vi "Append Text.vi"(7 "Style":T1={"Name"="Default", "Font"={"Name"="Calibri", "Size"=12, "Bold"=FALSE, "Italic"=FALSE, "Underline"=18, "Strike"=FALSE, "Color"=0, "Alignment"=1}} {"Font"."Alignment" items=["LEFT"=1, "CENTER"=2, "RIGHT"=3, "BOTH"=4, "MEDIUM_KASHIDA"=5, "DISTRIBUTE"=6, "NUM_TAB"=7, "HIGH_KASHIDA"=8, "LOW_KASHIDA"=9, "THAI_DISTRIBUTE"=10]; "Font"."Underline" items=["Single"=1, "Words"=2, "Double"=3, "Thick"=4, "Dotted"=5, "DottedHeavy"=6, "Dash"=7, "DashedHeavy"=8, "DashLong"=9, "DashLongHeavy"=10, "DotDash"=11, "DashDotHeavy"=12, "DotDotDash"=13, "DashDotDotHeavy"=14, "Wave"=15, "WavyHeavy"=16, "WavyDouble"=17, "None"=18]}, 8 "error in (no error)":errorcluster, 10 "Text":string, 11 "Document in":refnum<class "Document.lvclass">) -> (0 "error out":errorcluster, 3 "Document out":refnum<class "Document.lvclass">)   [LabVIEW 2017, in "LabVIEW NPOI.lvlib" / "Document.lvclass"]
uses:
  Document.lvclass
  Styles/Style--cluster.ctl
  Styles/Font--cluster.ctl
  Styles/Underline--ring.ctl
  Styles/Alignment--ring.ctl
  Styles/Styles.lvlib
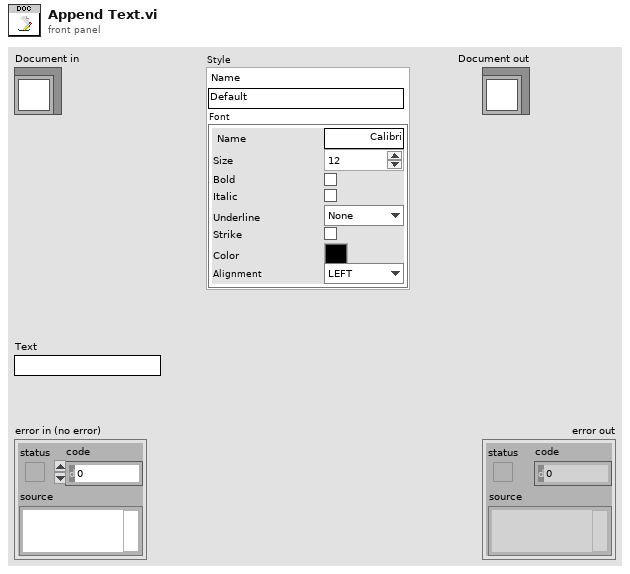
[diagram p1: front panel]
types:
  T1 = typedef "Styles.lvlib/Style--cluster.ctl" = cluster{"Name":string, "Font":T2}
  T2 = typedef "Styles.lvlib/Font--cluster.ctl" = cluster{"Name":string, "Size":i32, "Bold":bool, "Italic":bool, "Underline":T3, "Strike":bool, "Color":u32, "Alignment":T4}
  T3 = typedef "Styles.lvlib/Underline--ring.ctl" = i32
  T4 = typedef "Styles.lvlib/Alignment--ring.ctl" = i32
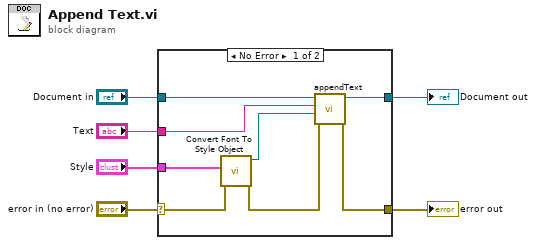
[diagram p0: block diagram]
diagram:
  n1 = case shown="No Error" "error in (no error)" {
    selector: "error in (no error)" -> [w9 w16]
    tunnel: [w7 w16] -> w5
    tunnel: [w12 w15] -> w3
    tunnel: "Document in" -> [w13 w15]
    tunnel: "Style" -> [w14 _]
    tunnel: "Text" -> [w10 _]
    frame No Error {
      n2 = call "Convert Font To Style Object.vi"("error in (no error)"=w9, "Style"=w14) -> ("error out"=w8:errorcluster, "Style Object"=w11:refnum<class "Style.lvclass">)  [unwired: 8 in]
      n3 = call-dynamic "appendText.vi"("error in (no error)"=w8, "Style"=w11, "Text"=w10, "Document in"=w13) -> ("error out"=w7:errorcluster, "Document out"=w12:refnum<class "Document.lvclass">)  [unwired: 6 in]
    }
    frame Error {
    }
  }
  "error out" <- w5
  "Document out" <- w3
